vi "题目5.vi"() -> ()   [LabVIEW 2017]
panel:
  in  "数值":dbl
  out "恭喜":bool
  out "通过":bool
  out "警告":bool
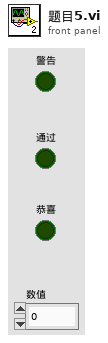
[diagram p1: front panel]
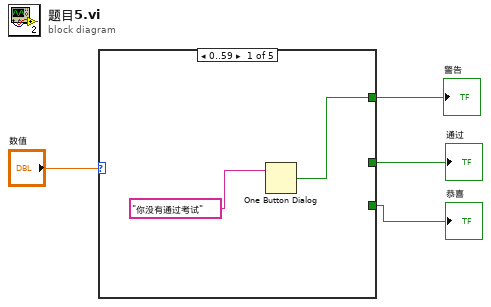
[diagram p0: block diagram]
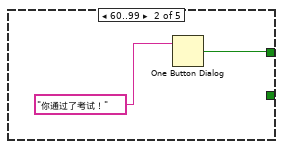
[diagram p2: hidden frame]
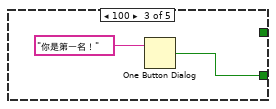
[diagram p3: hidden frame]
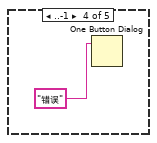
[diagram p4: hidden frame]
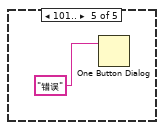
[diagram p5: hidden frame]
diagram:
  n1 = case shown="0..59" "数值" {
    tunnel: [_ w7 _ _ _] -> w3
    tunnel: [_ _ w9 _ _] -> w1
    tunnel: [w5 _ _ _ _] -> w2
    frame 0..59 {
      n2 = One Button Dialog(message="你没有通过考试" ("消息")) -> (true=w5:bool)  [unwired: 1 in]
    }
    frame 60..99 {
      n3 = One Button Dialog(message="你通过了考试！" ("消息")) -> (true=w7:bool)  [unwired: 1 in]
    }
    frame 100 {
      n4 = One Button Dialog(message="你是第一名！" ("消息")) -> (true=w9:bool)  [unwired: 1 in]
    }
    frame ..-1 {
      n5 = One Button Dialog(message="错误" ("消息")) -> ()  [unwired: 1 in, 1 out]
    }
    frame 101.. {
      n6 = One Button Dialog(message="错误" ("消息")) -> ()  [unwired: 1 in, 1 out]
    }
  }
  "警告" <- w2
  "通过" <- w3
  "恭喜" <- w1
